vi "stop daemon.vi"(8 "error in (no error)":errorcluster) -> (0 "error out":errorcluster)   [LabVIEW 2016, in "数据传输系统-05.lvlib" / "update.lvlib"]
uses:
  update.lvlib
panel:
  out "standard error":string caption="标准错误"
  out "standard output":string caption="标准输出"
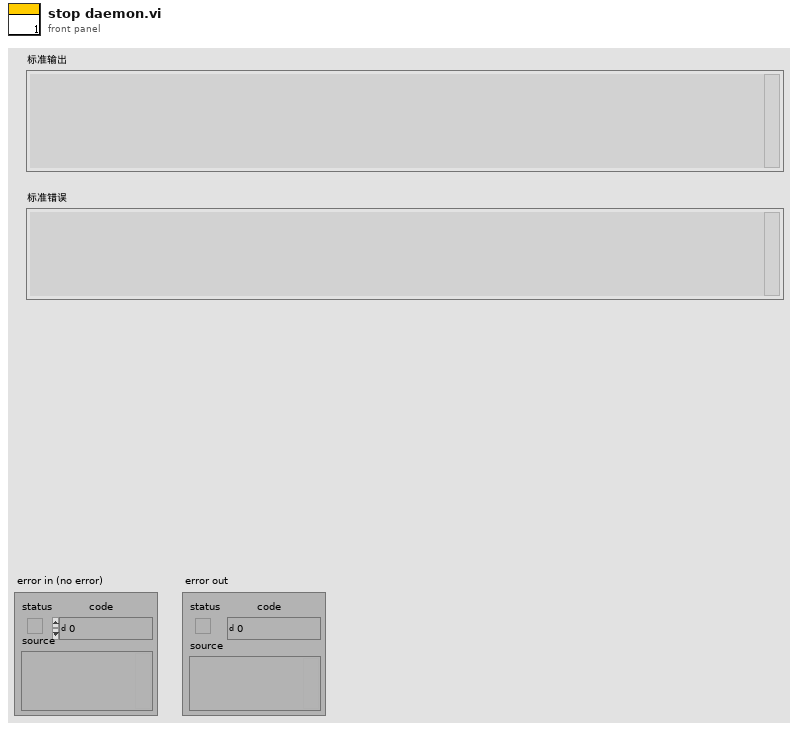
[diagram p1: front panel]
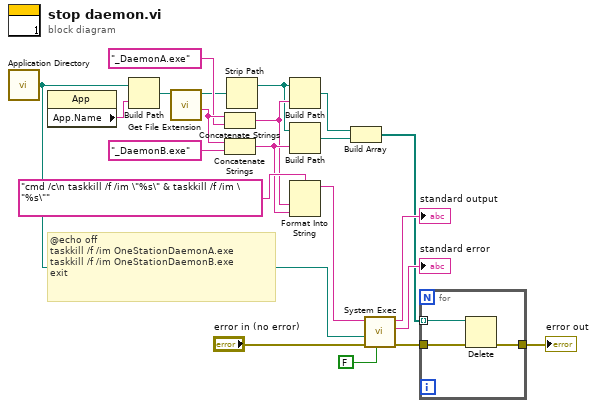
[diagram p0: block diagram]
diagram:
  # "@echo off\ntaskkill /f /im OneStationDaemonA.exe\ntaskkill /f /im OneStationDaemonB.exe\nexit"
  n1 = call <vilib>:"Application Directory.vi"() -> ("Application Directory"=w5:path)
  n2 = property class="App"() -> ("App.Name"=w15:string)  [unwired: 2 in, 2 out]
  n3 = Build Path(base path=w5, name or relative path=w15) -> (appended path=w14:path)
  n4 = call <vilib>:"Get File Extension.vi"("file"=w14) -> ("filename without extension"=w19:string, "dup file"=w12:path)  [unwired: 6 in, 3 out]
  n5 = Concatenate Strings(w19, "_DaemonA.exe" ("名称或相对路径")) -> (w10:string)
  n6 = Concatenate Strings(w19, "_DaemonB.exe" ("名称或相对路径")) -> (w11:string)
  n7 = Strip Path(path=w12) -> (stripped path=w7:path)  [unwired: 1 out]
  n8 = Build Path(base path=w7, name or relative path=w10) -> (appended path=w8:path)
  n9 = Build Path(base path=w7, name or relative path=w11) -> (appended path=w9:path)
  n10 = Format Into String(format string="cmd /c\n taskkill /f /im \"%s\" & taskkill /f /im \"%s\"" ("格式字符串"), w10, w11) -> (resulting string=w4:string)  [unwired: 2 in, 1 out]
  n11 = Build Array(w8, w9) -> (w3:path[])
  n12 = call <vilib>:"System Exec.vi"("run minimized? (F)"=FALSE, "error in (no error)"="error in (no error)", "working directory"=w5, "command line"=w4) -> ("error out"=w6:errorcluster, "standard error"=→"standard error":string, "standard output"=→"standard output":string)  [unwired: 4 in, 1 out]
  n13 = for {
    tunnel: w3 -> [w24] mode=indexing
    tunnel: w6 -> [w23]
    tunnel: [w22] -> w2
    n14 = Delete(path (use dialog)=w24, error in=w23) -> (error out=w22:errorcluster)  [unwired: 3 in, 2 out]
  }
  "error out" <- w2
